vi "Add DataTable Variable.vi"   [LabVIEW 2019, in "JMP Automation.lvlib"]
uses:
  <instrlib>/LV_JMP_bridge/JMP Automation.lvlib
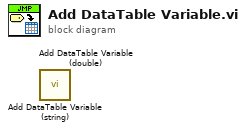
[diagram p0: block diagram]
diagram:
  n1 = call <instrlib>:"Add DataTable Variable (string).vi"() -> ()  [unwired: 10 in, 2 out]
  n2 = call <instrlib>:"Add DataTable Variable (double).vi"() -> ()  [unwired: 10 in, 2 out]
